vi "Arm Control.vi"(1 "Arm Control":dbl(slide) scale=-1.0..1.0) -> (0 "Setpoint angle":dbl)   [LabVIEW 2023]
uses:
  <vilib>/ptbypt/NI_PtbyPt.lvlib
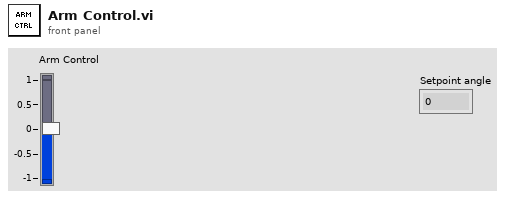
[diagram p1: front panel]
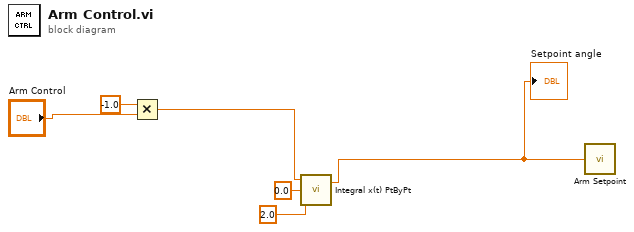
[diagram p0: block diagram]
diagram:
  n1 = Multiply(x=-1.0, y="Arm Control") -> (x*y=w4:dbl)
  n2 = call <vilib>:"Integral x(t) PtByPt.vi"("dt"=2.0, "initial condition"=0.0, "x"=w4) -> ("integral x(t)"=w1:dbl)  [unwired: 1 in, 1 out]
  "Setpoint angle" <- w1
  n3 = call "Arm Setpoint.vi"("Setpoint Angle"=w1) -> ()  [unwired: 1 in]
